vi "PQstatus.vi"(8 "error in (no error)":errorcluster, 11 "conn":u32) -> (0 "error out":errorcluster, 2 "PQStatus":T1(ring), 3 "conn out":u32)   [LabVIEW 2019, in "libpqlv.lvlib"]
uses:
  libpqlv.lvlib
  libpq.dll
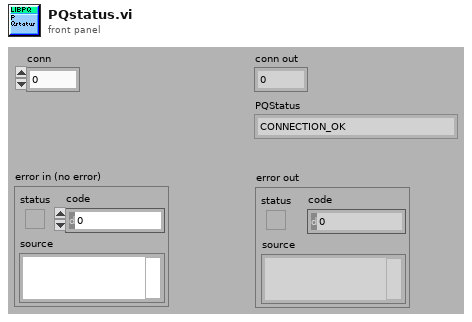
[diagram p1: front panel]
types:
  T1 = enum32{"CONNECTION_OK", "CONNECTION_BAD", "CONNECTION_STARTED", "CONNECTION_MADE", "CONNECTION_AWAITING_RESPONSE", "CONNECTION_AUTH_OK", "CONNECTION_SETENV", "CONNECTION_SSL_STARTUP", "CONNECTION_NEEDED"}
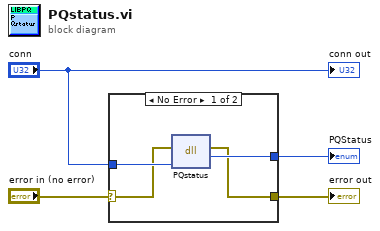
[diagram p0: block diagram]
diagram:
  n1 = case shown="No Error" "error in (no error)" {
    selector: "error in (no error)" -> [w6 w9]
    tunnel: [w5 w9] -> w3
    tunnel: [w8 _] -> w2
    tunnel: "conn" -> [w7 _]
    frame No Error {
      n2 = dll-call lib="libpq.*" fn="PQstatus"(error in=w6, "conn"=w7) -> (error out=w5:errorcluster, "PQstatus"=w8:u32)  [unwired: 3 in, 1 out]
    }
    frame Error {
    }
  }
  "error out" <- w3
  "PQStatus" <- w2
  "conn out" <- "conn"
